vi "ClusterLabels.vi"(11 "abc":refnum<vi>) -> (0 "Label.Text":string, 3 "Array":string[](array[string]))   [LabVIEW 2013, in "main.lvlib"]
uses:
  main.lvlib
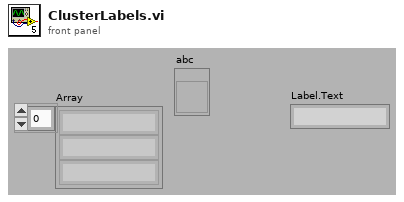
[diagram p1: front panel]
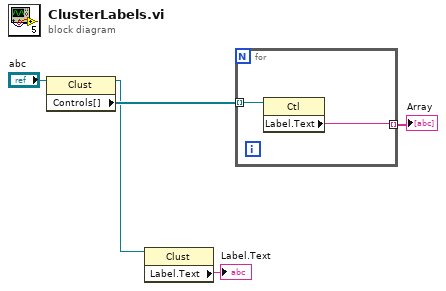
[diagram p0: block diagram]
diagram:
  n1 = property class="Clust"(reference="abc") -> (reference out=w3:refnum<vi>, "Controls[]"=w4:refnum<vi>[])  [unwired: 1 in, 1 out]
  n2 = property class="Clust"(reference=w3) -> ("Label.Text"=→"Label.Text":string)  [unwired: 1 in, 2 out]
  n3 = for {
    tunnel: [w7] -> w5 mode=indexing
    tunnel: w4 -> [w6] mode=indexing
    n4 = property class="Ctl"(reference=w6) -> ("Label.Text"=w7:string)  [unwired: 1 in, 2 out]
  }
  "Array" <- w5
